vi "Configure HVPS.vi"(8 "error in":errorcluster, 11 "Config Handle":T1) -> (0 "error out":errorcluster, 3 "Session HVPS out":refnum<class "Session HVPS.lvclass">)   [LabVIEW 2014, in "Session HVPS.lvclass"]
doc: "Check the HVPS key 'Type' to determine what the correct instance of the HVPS class is. Once the class has been determined, call the appropriate Configure method for that instance."
uses:
  Session Based/Base/Session HVPS.lvclass
  reusable/Session APIs/File Access/Config Data/Config Session.ctl
  reusable/Session APIs/File Access/Config Data/Config Data.lvclass
  reusable/Session APIs/File Access/Config Data/Config Data.lvclass/Config Data.ctl
  Configurable Device/Configurable Device.lvclass/Configurable Device.ctl
  reusable/Session APIs/File Access/Config Data/Accessors/Read Ref.vi
  Configurable Device/Write Handle.vi
  <vilib>/Utility/config.llb/Read Key (String).vi
  <vilib>/Utility/config.llb/NI_LVConfig.lvlib
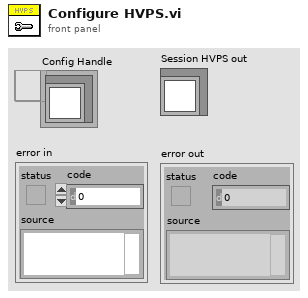
[diagram p1: front panel]
types:
  T1 = typedef "Config Data.lvclass/Config Session.ctl" = refnum<data-value>
  T2 = typedef "NI_LVConfig.lvlib/Config Data RefNum.ctl" = refnum<k1>
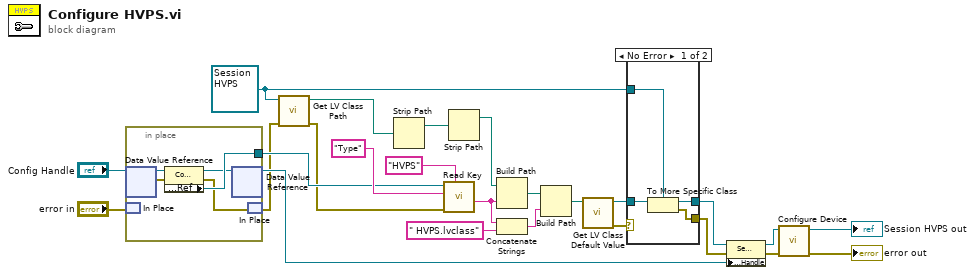
[diagram p0: block diagram]
diagram:
  w20 = refnum<class "Session HVPS.lvclass"> refnum ("Session HVPS out")
  n1 = in-place {
    in-place-border: [w28] -> w7
    n2 = in-place-dvr #1("Config Handle") -> (w30:refnum<class "Config Data.lvclass">, w29:errorcluster)
    n3 = in-place-match #2("error in") -> ()  [unwired: 1 out]
    n4 = property class="Config Data"(reference=w30, error in=w29) -> (reference out=w27:refnum<class "Config Data.lvclass">, error out=w26:errorcluster, "Accessors:Ref"=w28:T2)
    n5 = in-place-dvr #1(w27) -> (w6:T1)  [unwired: 1 out]
    n6 = in-place-match #2(w26) -> (w2:errorcluster)
  }
  n7 = call <vilib>:"Get LV Class Path.vi"("error in (no error)"=w2, "object"=w20) -> ("error out"=w1:errorcluster, "class path"=w8:path)  [unwired: 8 in]
  n8 = Strip Path(path=w8) -> (stripped path=w9:path)  [unwired: 1 out]
  n9 = call-poly <vilib>:"Read Key.vi"("section"="HVPS", "error in (no error)"=w1, "key"="Type", "refnum"=w7) -> ("value"=w14:string)  [unwired: 4 in, 3 out]
  n10 = Strip Path(path=w9) -> (stripped path=w12:path)  [unwired: 1 out]
  n11 = Build Path(base path=w12, name or relative path=w14) -> (appended path=w13:path)
  n12 = Concatenate Strings(w14, " HVPS.lvclass" ("string")) -> (w16:string)
  n13 = Build Path(base path=w13, name or relative path=w16) -> (appended path=w17:path)
  n14 = call <vilib>:"Get LV Class Default Value.vi"("class path"=w17) -> ("error out"=w18:errorcluster, "object"=w19:refnum<class>)  [unwired: 9 in]
  n15 = case shown="No Error" w18 {
    tunnel: w19 -> [w34 _]
    tunnel: w20 -> [w33 w35]
    tunnel: [w32 w35] -> w5
    tunnel: [w31 _] -> w3
    frame No Error {
      n16 = To More Specific Class(target class=w33, reference=w34) -> (specific class reference=w32:refnum<class "Session HVPS.lvclass">, error out=w31:errorcluster)  [unwired: 1 in]
    }
    frame Error {
    }
  }
  n17 = property class="Session HVPS"(reference=w5, error in=w3, "Accessors:Handle"=w6) -> (reference out=w24:refnum<class "Session HVPS.lvclass">, error out=w21:errorcluster)
  n18 = call-dynamic "Configure Device.vi"("error in"=w21, "Device in"=w24) -> ("error out"=→"error out":errorcluster, "Device out"=→"Session HVPS out":refnum<class "Session HVPS.lvclass">)  [unwired: 6 in, 2 out]
